vi "DAB Decode.vi"(11 "image data":T1) -> (3 "Message":string)   [LabVIEW 2020]
uses:
  <vilib>/picture/picture.llb/imagedata.ctl
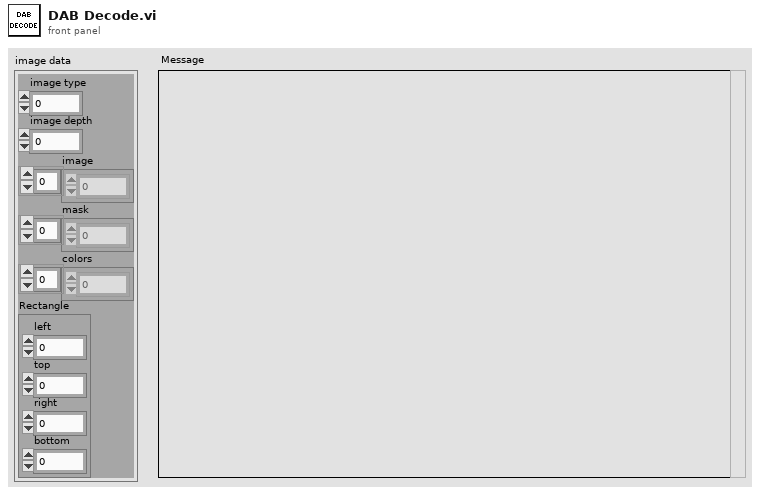
[diagram p1: front panel]
types:
  T1 = typedef "imagedata.ctl" = cluster{"image type":i32, "image depth":i32, "image":u8[], "mask":u8[], "colors":u32[], "Rectangle":cluster{"left":i16, "top":i16, "right":i16, "bottom":i16}}
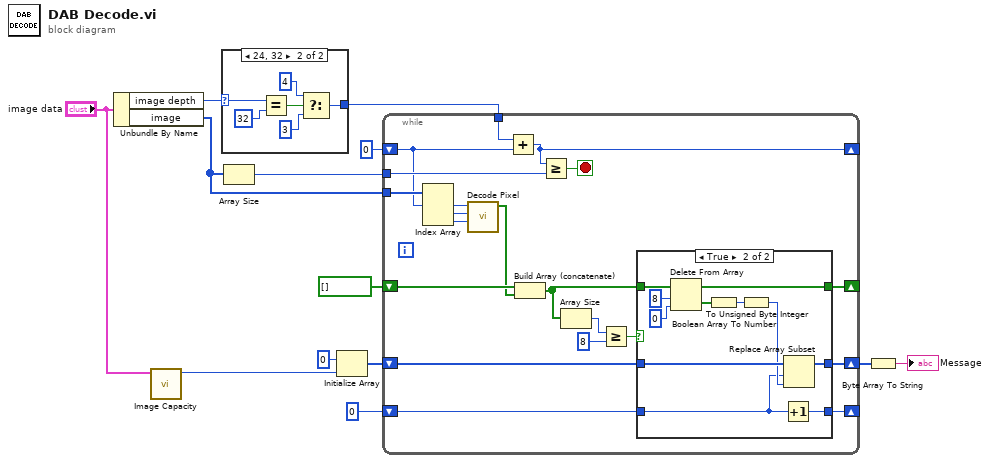
[diagram p0: block diagram]
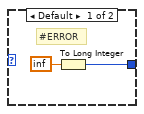
[diagram p2: hidden frame]
diagram:
  n1 = Unbundle By Name("image data") -> ("image depth"=w13:i32, "image"=w11:u8[])
  n2 = call "Image Capacity.vi"("image data"="image data") -> ("Capacity Bytes"=w1:i32)  [unwired: 10 in]
  n3 = case shown="24, 32" w13 {
    selector: w13 -> [_ w21]
    tunnel: [w14 w16] -> w10
    frame Default {
      # "#ERROR"
      n4 = To Long Integer(number=inf) -> (32bit integer=w14:i32)
    }
    frame 24, 32 {
      n5 = Equal?(x=w21, y=32) -> (x = y?=w19:bool)
      n6 = Select(t=4, s=w19, f=3) -> (s? t:f=w16:i32)
    }
  }
  n7 = Array Size(array=w11) -> (size(s)=w9:i32)
  n8 = Initialize Array(u8 0, w1) -> (w6:u8[])
  n9 = while {
    shift-right: [w41] -> _
    shift-left: 0 -> [w37]
    tunnel: w9 -> [w40]
    tunnel: w10 -> [w36]
    tunnel: w11 -> [w38]
    shift-right: [w26] -> _
    shift-left: bool[] [] -> [w32]
    shift-right: [w25] -> w4
    shift-left: w6 -> [w24]
    shift-right: [w23] -> _
    shift-left: 0 -> [w22]
    stop <- w39 stop-if-true
    n10 = Index Array(array=w38, index #1=w37) -> (element #1=w35:u8, element #2=w34:u8, element #3=w33:u8)  [unwired: 2 in]
    n11 = call "Decode Pixel.vi"("B"=w33, "G"=w34, "R"=w35) -> ("Bits"=w31:bool[])  [unwired: 8 in]
    n12 = Add(x=w36, y=w37) -> (x+y=w41:i32)
    n13 = Build Array (concatenate)(w32, w31) -> (w27:bool[])
    n14 = Greater Or Equal?(x=w41, y=w40) -> (x >= y?=w39:bool)
    n15 = Array Size(array=w27) -> (size(s)=w30:i32)
    n16 = Greater Or Equal?(x=w30, y=8) -> (x >= y?=w28:bool)
    n17 = case shown="True" w28 {
      tunnel: w27 -> [w44 w55]
      tunnel: [w44 w54] -> w26
      tunnel: [w43 w47] -> w25
      tunnel: w24 -> [w43 w50]
      tunnel: [w42 w45] -> w23
      tunnel: w22 -> [w42 w46]
      frame False {
      }
      frame True {
        n18 = Delete From Array(array=w55, length=8, index=0) -> (deleted portion=w51:bool[], array with subset deleted=w54:bool[])
        n19 = Boolean Array To Number(Boolean array=w51) -> (number=w49:u32)
        n20 = To Unsigned Byte Integer(number=w49) -> (unsigned 8bit integer=w48:u8)
        n21 = Increment(x=w46) -> (x+1=w45:i32)
        n22 = Replace Array Subset(array=w50, new element=w48, index=w46) -> (w47:u8[])
      }
    }
  }
  n23 = Byte Array To String(unsigned byte array=w4) -> (string=→"Message":string)
